vi "LineFollow_Step.vi"(2 "Pickup Distance":i32, 3 "Turn Speed":i32, 4 "Drive Speed":i32) -> (0 "Ultrasonic Distance":dbl, 1 "Object Detected":bool)   [LabVIEW 2016, in "Budda_V2.lvrbt"]
uses:
  Budda_V2.lvrbt
  <vilib>/NXT/Block Support/NXT_InputPort.ctl
  <vilib>/NXT/Subs/ColorSensorColors.ctl
  <vilib>/NXT/Block Support/NXT_OutputPort.ctl
  <vilib>/NXT/Dual Mode Library/Sensors/EV3_Color_Color.vi
  <vilib>/NXT/NXTIO Xnodes/NXTIONodeSubVIs/NXTMoveMotors.vi
  <vilib>/NXT/Dual Mode Library/Sensors/EV3_Ultrasonic_CM.vi
  <vilib>/NXT/Subs/LVHSConnector.ctl
  <vilib>/NXT/NXTIO Xnodes/AddressXNode/NXTIOAddress.xnode
  <vilib>/NXT/NXTIO Xnodes/NXTIOXNode/NXTIO.xnode
  <vilib>/NXT/LegoClasses/BrickReference/BrickReference.lvclass
panel:
  in  "stop":bool
  in  "-Turn Speed":dbl
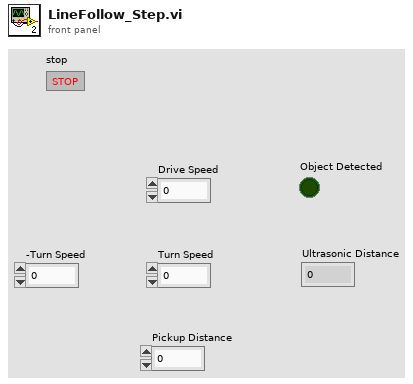
[diagram p1: front panel]
types:
  T1 = typedef "ColorSensorColors.ctl" = enum16{"No Color", "Black", "Blue", "Green", "Yellow", "Red", "White", "Brown"}
  T2 = typedef "NXT_InputPort.ctl" = u32
  T3 = typedef "NXT_OutputPort.ctl" = u8
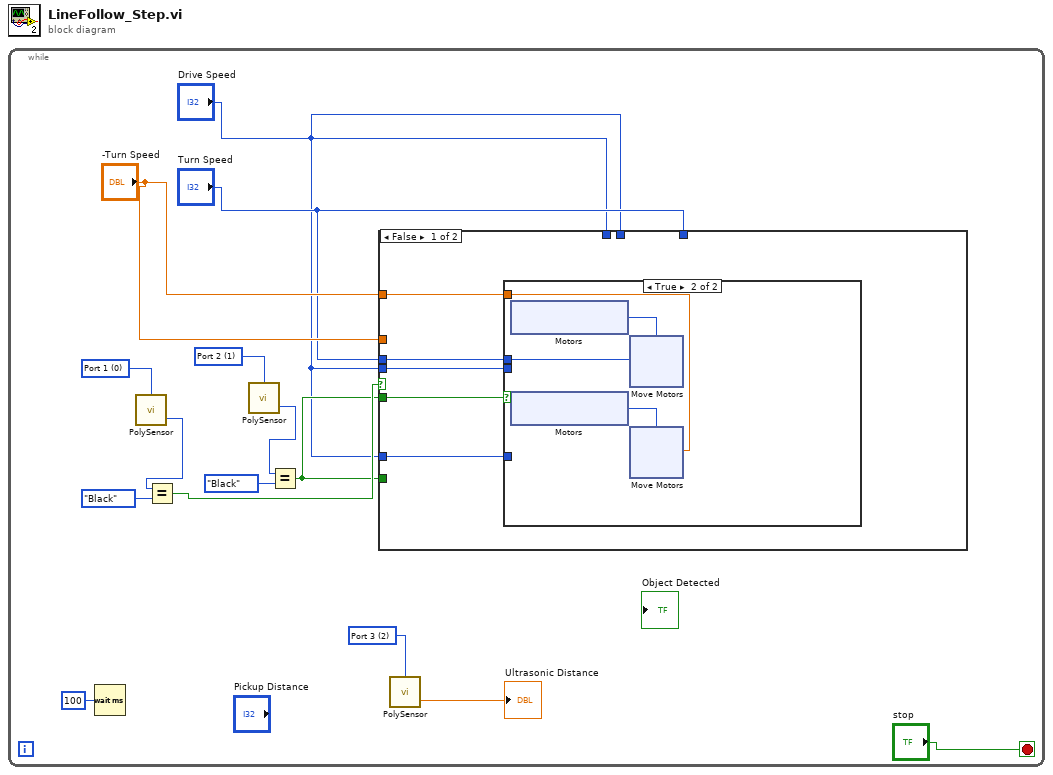
[diagram p0: block diagram]
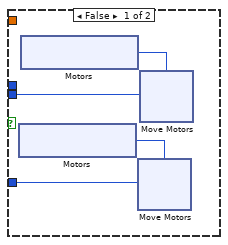
[diagram p2: hidden frame]
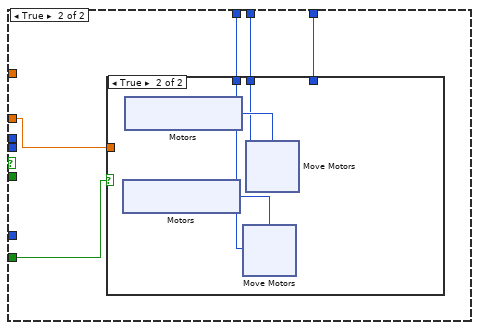
[diagram p3: hidden frame]
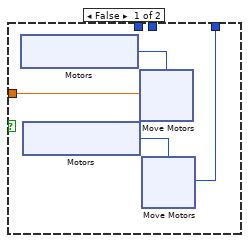
[diagram p4: hidden frame]
diagram:
  n1 = while {
    stop <- "stop" stop-if-true
    w2 = T2 2 items=["Port 1", "Port 2", "Port 3", "Port 4"] ("Port (Port 1)")
    w14 = T2 1 items=["Port 1", "Port 2", "Port 3", "Port 4"] ("Port (Port 1)")
    w15 = T2 0 items=["Port 1", "Port 2", "Port 3", "Port 4"] ("Port (Port 1)")
    n2 = Wait (ms)(milliseconds to wait=u32 100) -> ()  [unwired: 1 out]
    n3 = call-poly <vilib>:"PolySensor.vi"("Port (Port 1)"=w15) -> ("Detected Color"=w13:T1)  [unwired: 2 in, 1 out]
    n4 = Equal?(x=w13, y=ColorSensorColors."Black") -> (x = y?=w9:bool)
    n5 = call-poly <vilib>:"PolySensor.vi"("Port (Port 1)"=w14) -> ("Detected Color"=w12:T1)  [unwired: 2 in, 1 out]
    n6 = Equal?(x=w12, y=ColorSensorColors."Black") -> (x = y?=w8:bool)
    n7 = case shown="False" w9 {
      tunnel: w8 -> [w20 _]
      tunnel: "Drive Speed" -> [w19 _]
      tunnel: "Drive Speed" -> [w18 _]
      tunnel: "Turn Speed" -> [w17 _]
      tunnel: "-Turn Speed" -> [w16 _]
      tunnel: w8 -> [_ w65]
      tunnel: "-Turn Speed" -> [_ w64]
      tunnel: "Turn Speed" -> [_ w63]
      tunnel: "Drive Speed" -> [_ w62]
      tunnel: "Drive Speed" -> [_ w61]
      frame False {
        n8 = case shown="True" w20 {
          tunnel: w19 -> [w23 _]
          tunnel: w18 -> [w21 _]
          tunnel: w17 -> [_ w43]
          tunnel: w16 -> [_ w41]
          frame False {
            n9 = xnode "Motors"() -> ("Motor"=w22:T3)
            n10 = xnode "Motors"() -> ("Motor"=w24:T3)
            n11 = xnode "Move Motors"("Power/Speed 1"=w21, "Motors"=w22) -> ()  [unwired: 1 in, 1 out]
            n12 = xnode "Move Motors"("Power/Speed 1"=w23, "Motors"=w24) -> ()  [unwired: 1 in, 1 out]
          }
          frame True {
            n13 = xnode "Motors"() -> ("Motor"=w44:T3)
            n14 = xnode "Motors"() -> ("Motor"=w42:T3)
            n15 = xnode "Move Motors"("Power/Speed 1"=w43, "Motors"=w44) -> ()  [unwired: 1 in, 1 out]
            n16 = xnode "Move Motors"("Power/Speed 1"=w41, "Motors"=w42) -> ()  [unwired: 1 in, 1 out]
          }
        }
      }
      frame True {
        n17 = case shown="True" w65 {
          tunnel: w64 -> [w68 _]
          tunnel: w63 -> [w66 _]
          tunnel: w62 -> [_ w87]
          tunnel: w61 -> [_ w86]
          frame False {
            n18 = xnode "Motors"() -> ("Motor"=w69:T3)
            n19 = xnode "Motors"() -> ("Motor"=w67:T3)
            n20 = xnode "Move Motors"("Power/Speed 1"=w68, "Motors"=w69) -> ()  [unwired: 1 in, 1 out]
            n21 = xnode "Move Motors"("Power/Speed 1"=w66, "Motors"=w67) -> ()  [unwired: 1 in, 1 out]
          }
          frame True {
            n22 = xnode "Motors"() -> ("Motor"=w89:T3)
            n23 = xnode "Motors"() -> ("Motor"=w88:T3)
            n24 = xnode "Move Motors"("Power/Speed 1"=w86, "Motors"=w89) -> ()  [unwired: 1 in, 1 out]
            n25 = xnode "Move Motors"("Power/Speed 1"=w87, "Motors"=w88) -> ()  [unwired: 1 in, 1 out]
          }
        }
      }
    }
    n26 = call-poly <vilib>:"PolySensor.vi"("Port (Port 1)"=w2) -> ("Centimeters"=→"Ultrasonic Distance":sgl)  [unwired: 2 in, 1 out]
  }
